vi "DLL 사용.vi"() -> ()   [LabVIEW 2014]
panel:
  out "arrayOut":dbl[](array[numeric])
  in  "filePath":string="C:\\Users\\lvedu03\\Desktop\\중급 LV 실습\\DLL.txt"
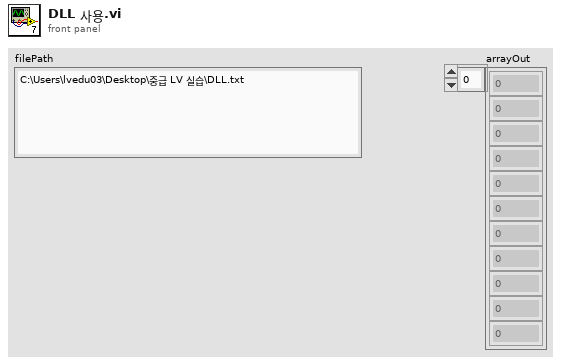
[diagram p1: front panel]
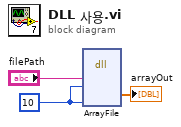
[diagram p0: block diagram]
diagram:
  w2 = 10 ("arraySize")
  n1 = dll-call lib="PTH2vabs CUserslvedu03Desktop중급 LV 실습builds공유라이브러리 만들기\n나의 DLL\nSharedLib.dll" fn="ArrayFile"("filePath"="filePath", "arraySize"=w2, "len"=w2) -> ("arrayOut"=→"arrayOut":dbl[])  [unwired: 8 in, 2 out]
